vi "titleAppend.vi"(10 "Final Title":string, 11 "String in":string) -> (3 "String out":string)   [LabVIEW 2012]
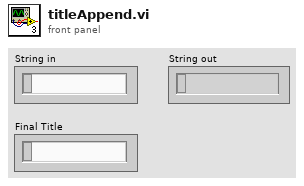
[diagram p1: front panel]
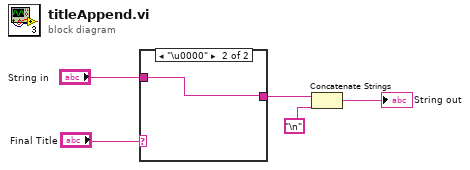
[diagram p0: block diagram]
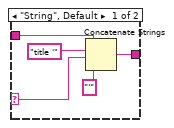
[diagram p2: hidden frame]
diagram:
  n1 = case shown="\"\"" "Final Title" {
    selector: "Final Title" -> [w6 _]
    tunnel: "String in" -> [w10 w11]
    tunnel: [w8 w11] -> w4
    frame "String", Default {
      n2 = Concatenate Strings(w10, "title '", w6, "'" ("string")) -> (w8:string)
    }
    frame "\u0000" {
    }
  }
  n3 = Concatenate Strings(w4, "\n") -> (→"String out":string)
